vi "Alt Trigger Demo.vi"() -> ()   [LabVIEW 2012]
panel:
  out "Alt Diff Down":bool
  out "Alt Dif Last":dbl
  out "Alt States":T1={"Main"=TRUE, "Boost A"=FALSE, "Boost B"=FALSE, "Recirc"=FALSE, "Scrubber"=FALSE, "O2 Valve"=FALSE, "Vent"=FALSE, "Alarm"=FALSE}
  in  "Alt Dif":dbl(slide) scale=-1000.0..1000.0
  in  "Stop Progam":bool
  out "Loops":i32
  in  "Alt Trigger":T2={"Boost A Hi"=0.0, "Boost A Lo"=-250.0, "Boost B Hi"=50.0, "Boost B Lo"=-150.0, "O2 Hi"=250.0, "O2 Lo"=400.0, "Vent Hi"=50.0, "Vent Lo"=200.0, "Recirc Hi"=50.0, "Recirc  Lo``"=-150.0}
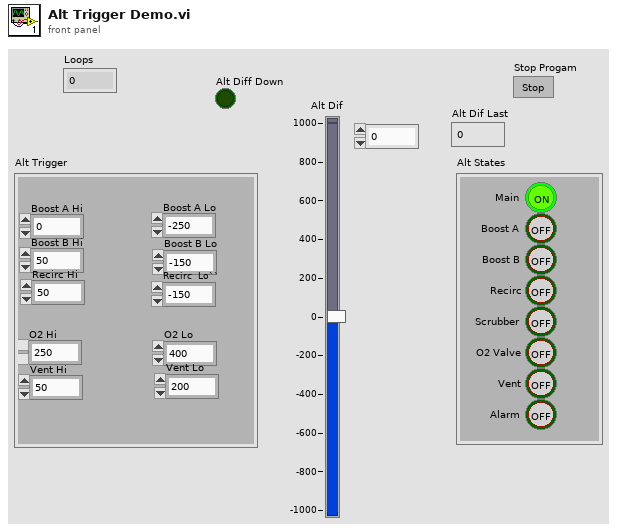
[diagram p1: front panel]
types:
  T1 = cluster{"Main":bool, "Boost A":bool, "Boost B":bool, "Recirc":bool, "Scrubber":bool, "O2 Valve":bool, "Vent":bool, "Alarm":bool}
  T2 = cluster{"Boost A Hi":dbl, "Boost A Lo":dbl, "Boost B Hi":dbl, "Boost B Lo":dbl, "O2 Hi":dbl, "O2 Lo":dbl, "Vent Hi":dbl, "Vent Lo":dbl, "Recirc Hi":dbl, "Recirc  Lo``":dbl}
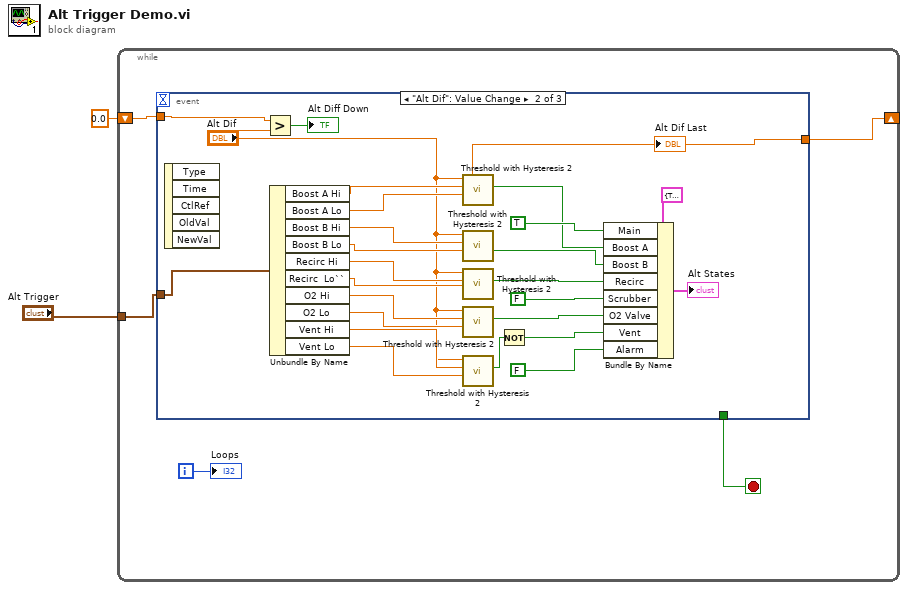
[diagram p0: block diagram]
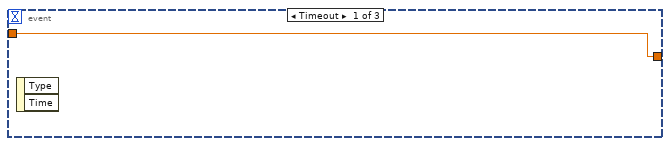
[diagram p2: hidden frame]
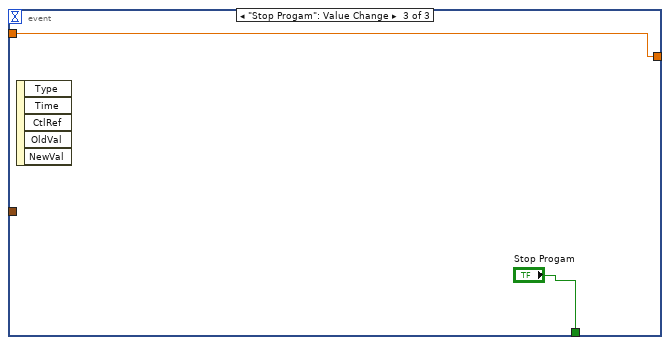
[diagram p3: hidden frame]
diagram:
  n1 = while {
    tunnel: "Alt Trigger" -> [w7]
    shift-right: [w4] -> _
    shift-left: 0.0 ("Out Dif Last") -> [w5]
    i -> [w6]
    stop <- w3 stop-if-true
    n2 = event shown="[1] \"Alt Dif\": Value Change" {
      selector: _ -> [_ _ _]
      dyn-events: _ -> [_ _ _]
      timeout: _ -> [_ _ _]
      tunnel: w7 -> [_ w9 _]
      tunnel: w5 -> [w8 w10 w36]
      tunnel: [w8 w11 w36] -> w4
      tunnel: [_ _ "Stop Progam"] -> w3
      event Timeout {
        n3 = event-data() -> ()  [unwired: 1 in, 2 out]
      }
      event "Alt Dif": Value Change {
        n4 = event-data() -> ()  [unwired: 1 in, 5 out]
        n5 = Greater?(x=w10, y="Alt Dif") -> (0:→"Alt Diff Down":bool)
        n6 = Unbundle By Name(w9) -> ("Boost A Hi"=w28:dbl, "Boost A Lo"=w27:dbl, "Boost B Hi"=w20:dbl, "Boost B Lo"=w21:dbl, "Recirc Hi"=w22:dbl, "Recirc  Lo``"=w23:dbl, "O2 Hi"=w17:dbl, "O2 Lo"=w16:dbl, "Vent Hi"=w25:dbl, "Vent Lo"=w24:dbl)
        n7 = call "Threshold with Hysteresis 2.vi"("Hystersis"=w27, "Threshold"=w28, "Input Dif"="Alt Dif") -> ("Power"=w15:bool, "Out Dif Last"=w11:dbl)  [unwired: 2 in, 2 out]
        "Alt Dif Last" <- w11
        n8 = call "Threshold with Hysteresis 2.vi"("Hystersis"=w21, "Threshold"=w20, "Input Dif"="Alt Dif") -> ("Threshold"=w26:bool)  [unwired: 2 in, 3 out]
        n9 = call "Threshold with Hysteresis 2.vi"("Hystersis"=w23, "Threshold"=w22, "Input Dif"="Alt Dif") -> ("Power"=w19:bool)  [unwired: 2 in, 3 out]
        n10 = call "Threshold with Hysteresis 2.vi"("Hystersis"=w16, "Threshold"=w17, "Input Dif"="Alt Dif") -> ("Power"=w18:bool)  [unwired: 2 in, 3 out]
        n11 = call "Threshold with Hysteresis 2.vi"("Hystersis"=w24, "Threshold"=w25, "Input Dif"="Alt Dif") -> ("Power"=w14:bool)  [unwired: 2 in, 3 out]
        n12 = Not(x=w14) -> (.not. x?=w29:bool)
        n13 = Bundle By Name(cluster=T1 {"Main"=TRUE, "Boost A"=FALSE, "Boost B"=FALSE, "Recirc"=FALSE, "Scrubber"=FALSE, "O2 Valve"=FALSE, "Vent"=FALSE, "Alarm"=FALSE} ("Alt States"), "Main"=TRUE, "Boost A"=w15, "Boost B"=w26, "Recirc"=w19, "Scrubber"=FALSE, "O2 Valve"=w18, "Vent"=w29, "Alarm"=FALSE) -> (→"Alt States":T1)
      }
      event "Stop Progam": Value Change {
        n14 = event-data() -> ()  [unwired: 1 in, 5 out]
      }
    }
    "Loops" <- w6
  }
